vi "Self Test.vi"(8 "error in":errorcluster, 11 "5105 in":refnum<class "5105.lvclass">) -> (0 "error out":errorcluster, 2 "Self Test Pass?":bool, 3 "5105 out":refnum<class "5105.lvclass">)   [LabVIEW 2019, in "5105.lvlib" / "5105.lvclass"]
uses:
  5105.lvclass
  Accessors/Read Local Resource.vi
  Accessors/Write Local Resource.vi
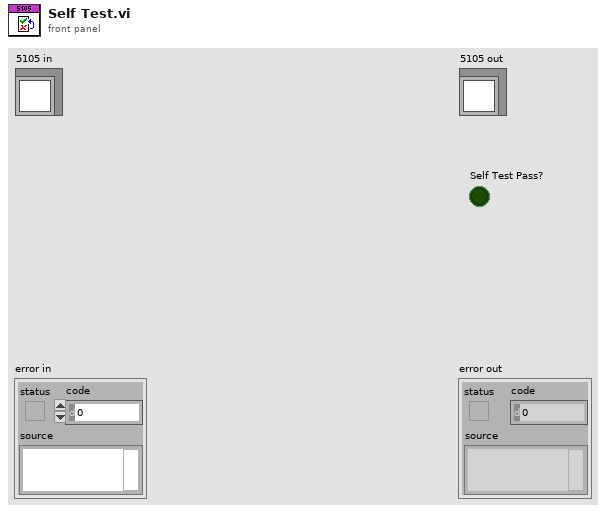
[diagram p1: front panel]
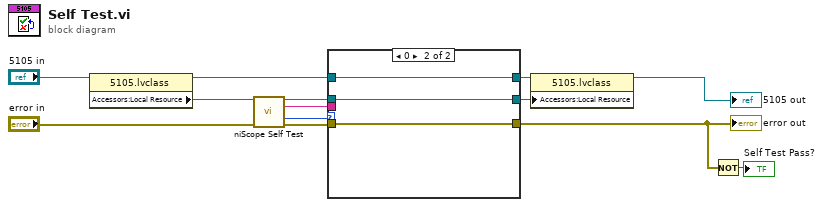
[diagram p0: block diagram]
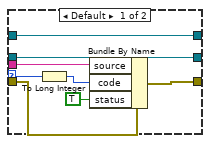
[diagram p2: hidden frame]
diagram:
  n1 = property class="5105.lvclass"(reference="5105 in") -> (reference out=w7:refnum<class "5105.lvclass">, "Accessors:Local Resource"=w8:refnum<k15>)  [unwired: 1 in, 1 out]
  n2 = call <instrlib>:"niScope Self Test.vi"("instrument handle"=w8, "error in"="error in") -> ("instrument handle out"=w6:refnum<k15>, "self-test message"=w3:string, "self test result"=w4:i16, "error out"=w5:errorcluster)  [unwired: 10 in]
  n3 = case shown="0" w4 {
    selector: w4 -> [w16 _]
    tunnel: w6 -> [w18 w23]
    tunnel: w5 -> [w21 w24]
    tunnel: w3 -> [w17 _]
    tunnel: [w19 w24] -> w12
    tunnel: [w18 w23] -> w2
    tunnel: w7 -> [w14 w22]
    tunnel: [w14 w22] -> w1
    frame Default {
      n4 = To Long Integer(number=w16) -> (32bit integer=w15:i32)
      n5 = Bundle By Name(cluster=w21, "source"=w17, "code"=w15, "status"=TRUE) -> (w19:errorcluster)
    }
    frame 0 {
    }
  }
  "error out" <- w12
  n6 = property class="5105.lvclass"(reference=w1, "Accessors:Local Resource"=w2) -> (reference out=→"5105 out":refnum<class "5105.lvclass">)  [unwired: 1 in, 1 out]
  n7 = Not(x=w12) -> (.not. x?=→"Self Test Pass?":bool)
